vi "Format JSON.vi"(6 "Variant in":variant, 7 "Shift Pressed?":bool, 8 "error in (no error)":errorcluster, 10 "QD Combo Box Ref":refnum<vi>, 11 "QD Launch VI Ref":refnum<vi>) -> (0 "error out":errorcluster, 4 "Variant out":variant)   [LabVIEW 2023]
doc: "This QuickDrop Plug-In formats a JSON String.\n\nDefault Shortcut - [F]"
uses:
  <vilib>/JDP Science/JSONtext/JSONtext.lvlib
panel:
  in  "Undo Name":string="Quick Drop Keyboard Shortcut"
  # "Do not change the connector pane of this VI.\n\nSee the block diagram for directions on how to use this template."
  # "Specify the name of the Undo transaction"
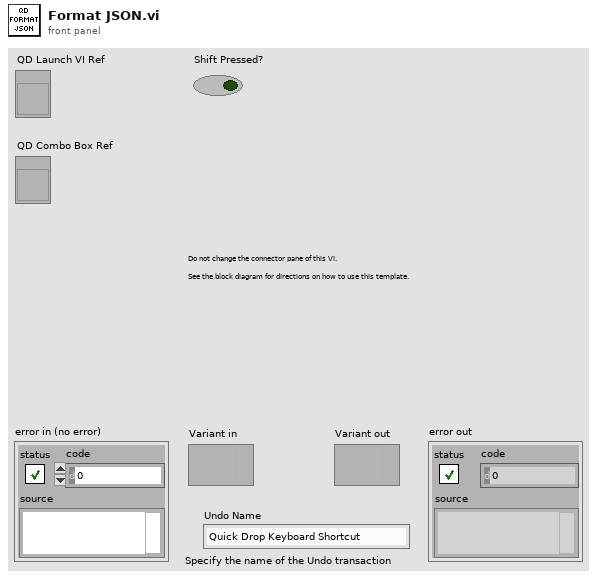
[diagram p1: front panel]
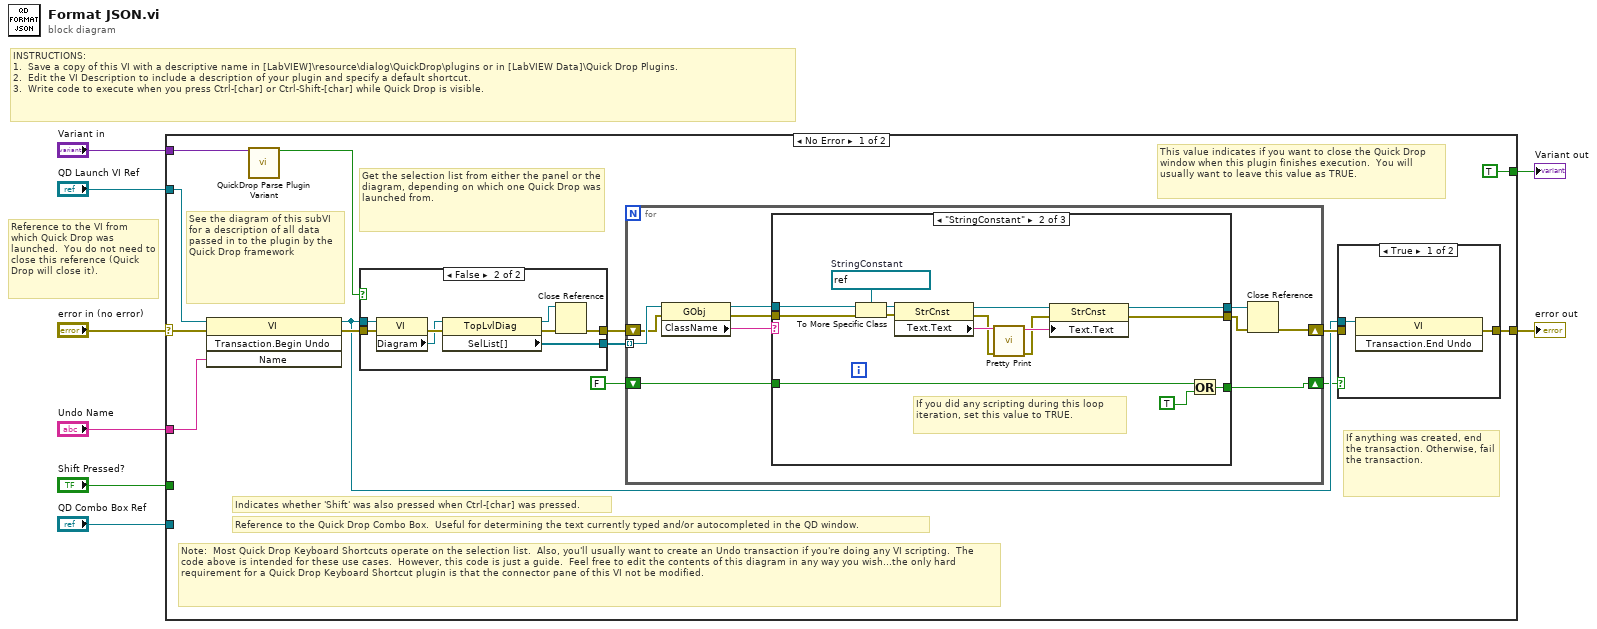
[diagram p0: block diagram]
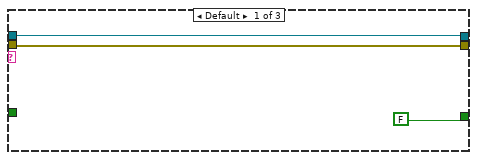
[diagram p2: hidden frame]
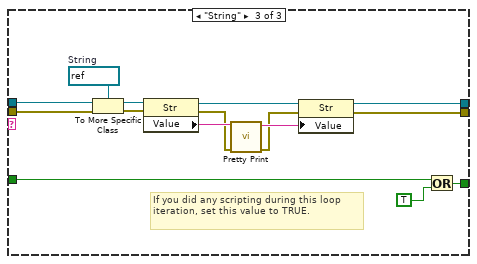
[diagram p3: hidden frame]
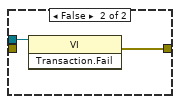
[diagram p4: hidden frame]
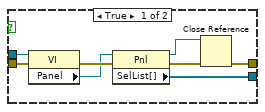
[diagram p5: hidden frame]
diagram:
  # "Reference to the VI from which Quick Drop was launched.  You do not need to close this reference (Quick Drop will close it)."
  # "INSTRUCTIONS:\n1.  Save a copy of this VI with a descriptive name in [LabVIEW]\\resource\\dialog\\QuickDrop\\plugins or in [LabVIEW Data]\\Quick Drop Plugins.\n2.  Edit the VI Description to include a description of your plugin and specify a default shortcut. \n3.  Write code to execute when you press Ctrl-[char] or Ctrl-Shift-[char] while Quick Drop is visible."
  n1 = case shown="No Error" "error in (no error)" {
    selector: "error in (no error)" -> [w21 w86]
    tunnel: [w15 w86] -> w7
    tunnel: "QD Launch VI Ref" -> [w20 _]
    tunnel: "Shift Pressed?" -> [_ _]
    tunnel: "QD Combo Box Ref" -> [_ _]
    tunnel: "Variant in" -> [w22 _]
    tunnel: "Undo Name" -> [w19 _]
    tunnel: [TRUE _] -> w1
    frame No Error {
      # "Note:  Most Quick Drop Keyboard Shortcuts operate on the selection list.  Also, you'll usually want to create an Undo transaction if you're doing any VI scripting.  The code above is intended for these use cases.  However, this code is just a guide.  Feel free to edit the contents of this diagram in any way you wish...the only hard requirement for a Quick Drop Keyboard Shortcut plugin is that the connector pane of this VI not be modified."
      # "Get the selection list from either the panel or the diagram, depending on which one Quick Drop was launched from."
      # "If anything was created, end the transaction. Otherwise, fail the transaction."
      # "This value indicates if you want to close the Quick Drop window when this plugin finishes execution.  You will usually want to leave this value as TRUE."
      # "See the diagram of this subVI for a description of all data passed in to the plugin by the Quick Drop framework"
      # "Reference to the Quick Drop Combo Box.  Useful for determining the text currently typed and/or autocompleted in the QD window."
      # "Indicates whether 'Shift' was also pressed when Ctrl-[char] was pressed."
      n2 = invoke class="VI" method="Transaction.Begin Undo"(reference=w20, error in=w21, "Name"=w19) -> (reference out=w12:refnum<vi>, error out=w16:errorcluster)  [unwired: 1 in, 2 out]
      n3 = call <vilib>:"QuickDrop Parse Plugin Variant.vi"("QDKS Variant in"=w22) -> ("QD Launch VI Panel?"=w17:bool)  [unwired: 12 in, 2 out]
      n4 = case shown="False" w17 {
        tunnel: w16 -> [w77 w85]
        tunnel: w12 -> [w76 w84]
        tunnel: [w71 w79] -> w14
        tunnel: [w70 w78] -> w9
        frame True {
          n5 = property class="VI"(reference=w76, error in=w77) -> (error out=w75:errorcluster, "Panel"=w74:refnum<vi>)  [unwired: 1 out]
          n6 = property class="Pnl"(reference=w74, error in=w75) -> (reference out=w72:refnum<vi>, error out=w73:errorcluster, "SelList[]"=w70:refnum<vi>[])
          n7 = Close Reference(reference=w72, error in (no error)=w73) -> (error out=w71:errorcluster)
        }
        frame False {
          n8 = property class="VI"(reference=w84, error in=w85) -> (error out=w83:errorcluster, "Diagram"=w82:refnum<vi>)  [unwired: 1 out]
          n9 = property class="TopLvlDiag"(reference=w82, error in=w83) -> (reference out=w80:refnum<vi>, error out=w81:errorcluster, "SelList[]"=w78:refnum<vi>[])
          n10 = Close Reference(reference=w80, error in (no error)=w81) -> (error out=w79:errorcluster)
        }
      }
      n11 = for {
        shift-right: [w23] -> w13
        shift-left: w14 -> [w28]
        shift-right: [w31] -> w10
        shift-left: FALSE -> [w32]
        tunnel: w9 -> [w30] mode=indexing
        n12 = property on="Property Node" class="GObj"(reference=w30, error in=w28) -> (reference out=w29:refnum<vi>, error out=w27:errorcluster, "ClassName"=w26:string)
        n13 = case shown="\"StringConstant\"" w26 {
          tunnel: w32 -> [_ w50 w65]
          tunnel: [FALSE w49 w64] -> w31
          tunnel: w29 -> [w34 w39 w54]
          tunnel: w27 -> [w33 w38 w53]
          tunnel: [w33 w36 w52] -> w25
          tunnel: [w34 w37 w51] -> w24
          frame Default {
          }
          frame "StringConstant" {
            w46 = refnum<vi> refnum  # StringConstant
            # "If you did any scripting during this loop iteration, set this value to TRUE."
            n14 = To More Specific Class(target class=w46, reference=w39, error in=w38) -> (specific class reference=w47:refnum<vi>, error out=w40:errorcluster)
            n15 = property on="Property Node" class="StrCnst"(reference=w47, error in=w40) -> (reference out=w45:refnum<vi>, error out=w41:errorcluster, "Text.Text"=w44:string)
            n16 = call <vilib>:"Pretty Print.vi"("error in (no error)"=w41, "JSON"=w44) -> ("error out"=w42:errorcluster, "<JSON>"=w43:string)  [unwired: 7 in, 1 out]
            n17 = property on="Property Node" class="StrCnst"(reference=w45, error in=w42, "Text.Text"=w43) -> (reference out=w37:refnum<vi>, error out=w36:errorcluster)
            n18 = Or(x=w50, y=TRUE ("x")) -> (x .or. y?=w49:bool)
          }
          frame "String" {
            w61 = refnum<vi> refnum  # String
            # "If you did any scripting during this loop iteration, set this value to TRUE."
            n19 = To More Specific Class(target class=w61, reference=w54, error in=w53) -> (specific class reference=w62:refnum<vi>, error out=w55:errorcluster)
            n20 = property on="Property Node" class="Str"(reference=w62, error in=w55) -> (reference out=w60:refnum<vi>, error out=w56:errorcluster, "Value"=w59:string)
            n21 = call <vilib>:"Pretty Print.vi"("error in (no error)"=w56, "JSON"=w59) -> ("error out"=w57:errorcluster, "<JSON>"=w58:string)  [unwired: 7 in, 1 out]
            n22 = property on="Property Node" class="Str"(reference=w60, error in=w57, "Value"=w58) -> (reference out=w51:refnum<vi>, error out=w52:errorcluster)
            n23 = Or(x=w65, y=TRUE ("x")) -> (x .or. y?=w64:bool)
          }
        }
        n24 = Close Reference(reference=w24, error in (no error)=w25) -> (error out=w23:errorcluster)
      }
      n25 = case shown="True" w10 {
        tunnel: w12 -> [w66 w68]
        tunnel: [w67 w69] -> w15
        tunnel: w13 -> [_ _]
        frame True {
          n26 = invoke class="VI" method="Transaction.End Undo"(reference=w66) -> (error out=w67:errorcluster)  [unwired: 2 in, 2 out]
        }
        frame False {
          n27 = invoke class="VI" method="Transaction.Fail"(reference=w68) -> (error out=w69:errorcluster)  [unwired: 2 in, 2 out]
        }
      }
    }
    frame Error {
    }
  }
  "error out" <- w7
  "Variant out" <- w1
